vi "PXI-Set DO Config.vi"(0 "DO Channels":i32[](array[numeric]), 5 "Sampling Rate (Hz)":dbl, 7 "Buffer Size":i32, 11 "error in (no error)":errorcluster) -> (15 "error out":errorcluster)   [LabVIEW 2020]
uses:
  DAQ Engine VIs/PXI Globals.vi
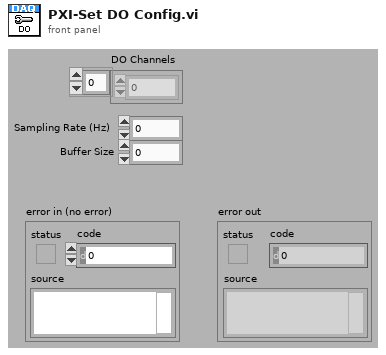
[diagram p1: front panel]
types:
  T1 = typedef "DI Channel Struct.ctl" = cluster{"Physical Channel":tag, "Channel Num":i32[]}
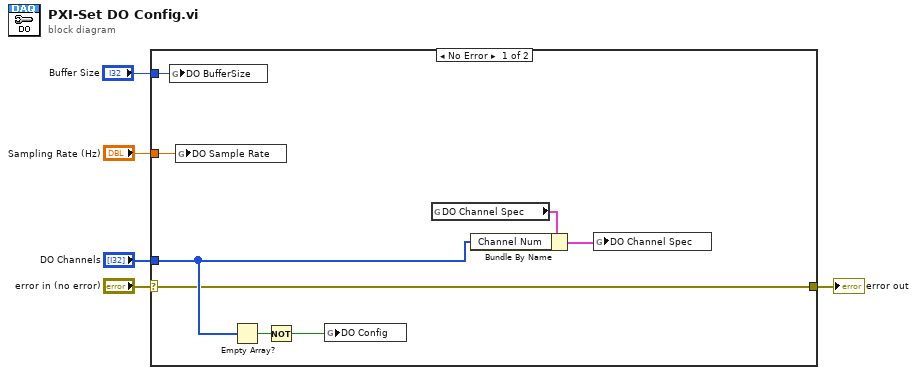
[diagram p0: block diagram]
diagram:
  n1 = case shown="No Error" "error in (no error)" {
    selector: "error in (no error)" -> [w6 w14]
    tunnel: "Sampling Rate (Hz)" -> [w12 _]
    tunnel: "DO Channels" -> [w8 _]
    tunnel: "Buffer Size" -> [w13 _]
    tunnel: [w6 w14] -> w1
    frame No Error {
      n2 = global write "PXI Globals.vi" "DO BufferSize"(w13) -> ()
      n3 = global write "PXI Globals.vi" "DO Sample Rate"(w12) -> ()
      n4 = Empty Array?(array=w8) -> (empty?=w11:bool)
      n5 = Not(x=w11) -> (.not. x?=w10:bool)
      n6 = global write "PXI Globals.vi" "DO Config"(w10) -> ()
      n7 = global read "PXI Globals.vi" "DO Channel Spec"() -> (w9:T1)
      n8 = Bundle By Name(cluster=w9, "Channel Num"=w8) -> (w7:T1)
      n9 = global write "PXI Globals.vi" "DO Channel Spec"(w7) -> ()
    }
    frame Error {
    }
  }
  "error out" <- w1
